vi "Logging Group Page.vi"(8 "error in (no error)":errorcluster, 11 "Node Ptr":T1 format="%.0x") -> (0 "error out":errorcluster)   [LabVIEW 2012, in "Waveform Data Logger System Explorer.lvlib"]
uses:
  Waveform Data Logger System Explorer.lvlib
  <vilib>/NI Veristand/Custom Device API/Custom Device Item Ref.ctl
  NationalInstruments.VeriStand.SystemDefinitionAPI
  NationalInstruments.VeriStand.SystemStorage
  Shared/Globals/Global GUIDs.vi
  <vilib>/NI Veristand/Custom Device Tools/Custom Device Utility Library/NI VeriStand - Search for All Items by GUID.vi
  <vilib>/NI VeriStand/Custom Device API/Custom Device API.lvlib
  <vilib>/NI VeriStand/Custom Device Tools/Custom Device Utility Library/Custom Device Utility Library.lvlib
  Shared/Waveform Data Logger Shared.lvlib
panel:
  in  "Description":string
  in  "Down Arrow":bool
  in  "Up Arrow":bool
  in  "Header 2":cluster{"Section Name":string}={"Section Name"="Waveform Log Files"}
  in  "Remove":bool
  in  "TDMS Log Files":i32(listbox)
  in  "Add File":bool
  in  "Header":cluster{"Section Name":string}={"Section Name"="Logging Group Specification"}
  in  "Name":string
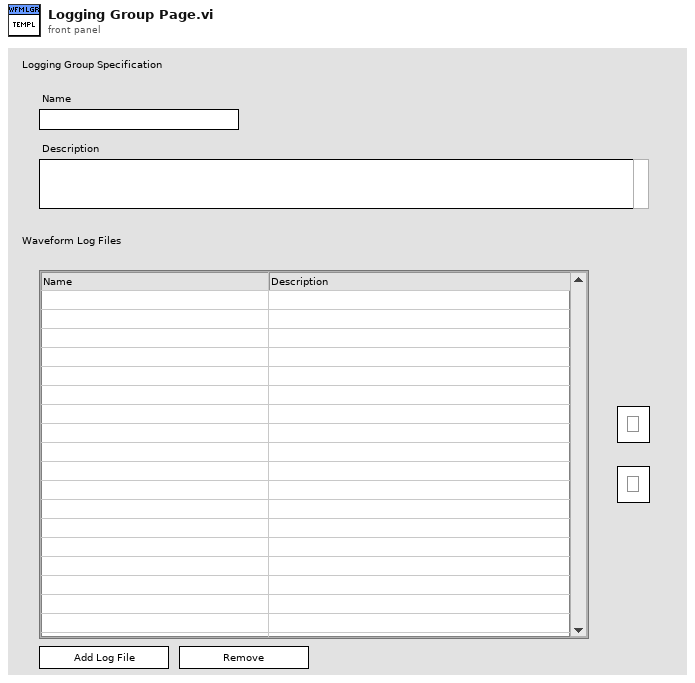
[diagram p1: front panel]
types:
  T1 = typedef "Custom Device API.lvlib/Custom Device Item Ref.ctl" = u64
  T2 = typedef "Custom Device API.lvlib/Custom Device Item Info.ctl" = cluster{"Name":string, "Is Channel":bool, "GUID":string, "Is Waveform":bool}
  T3 = typedef "Custom Device API.lvlib/Custom Device Commands.ctl" = enum16{"Default", "Item renamed", "Shutdown", "Dynamic button pressed"}
  T4 = typedef "LVRowAndColumnTypeDef.ctl" = cluster{"Row":i32, "Column":i32}
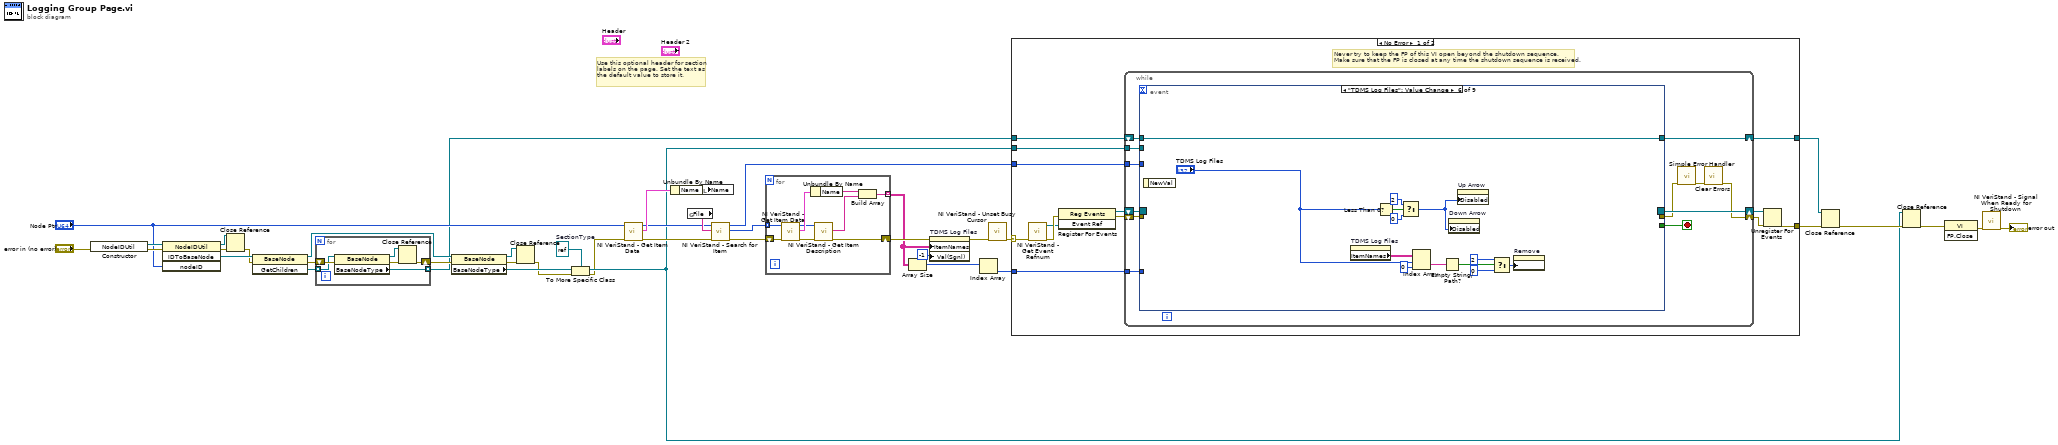
[diagram p0: block diagram]
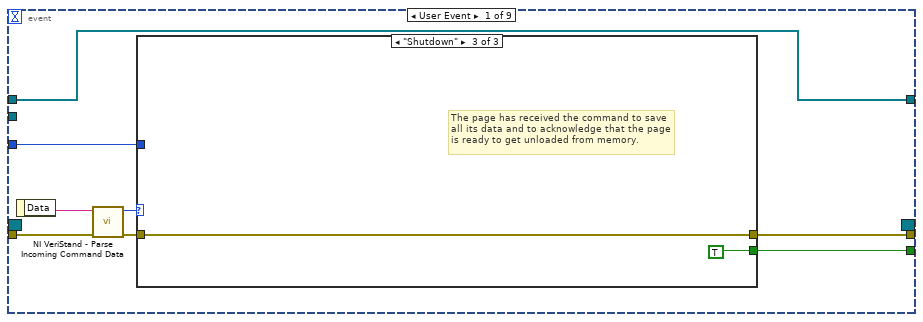
[diagram p2: hidden frame]
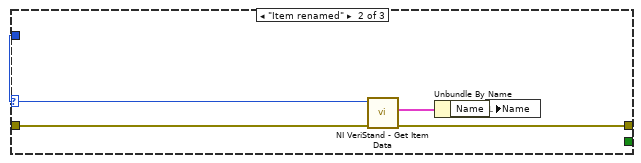
[diagram p4: hidden frame]
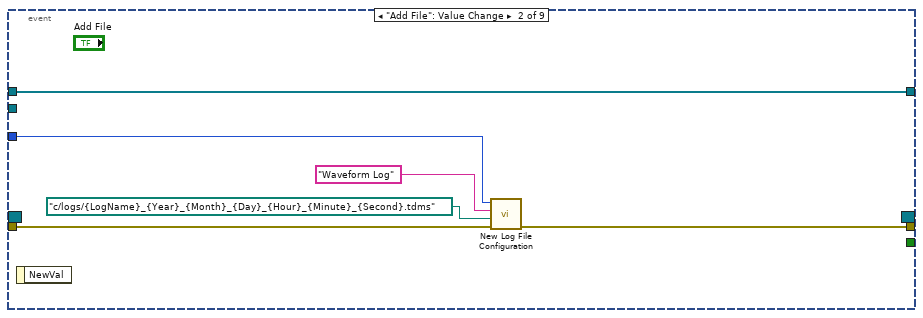
[diagram p5: hidden frame]
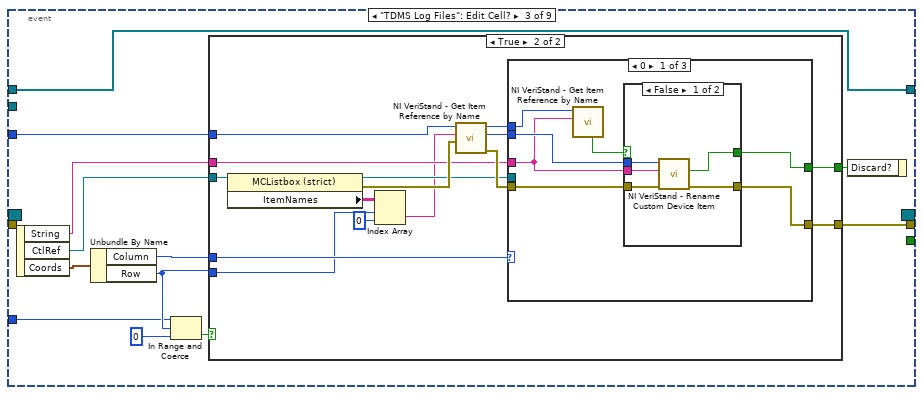
[diagram p6: hidden frame]
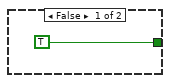
[diagram p7: hidden frame]
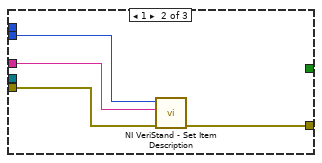
[diagram p9: hidden frame]
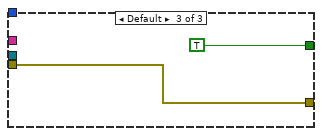
[diagram p10: hidden frame]
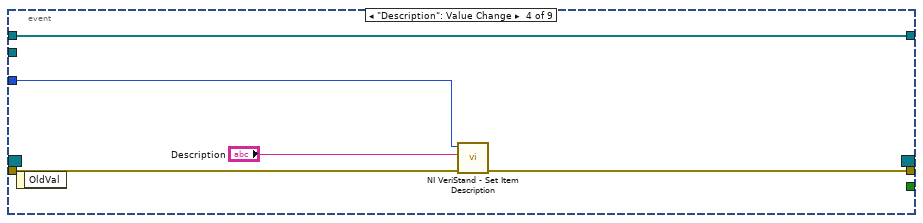
[diagram p11: hidden frame]
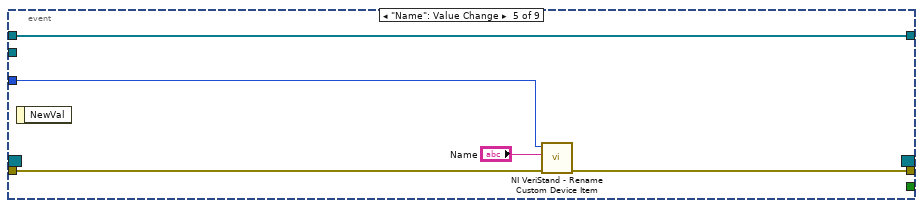
[diagram p12: hidden frame]
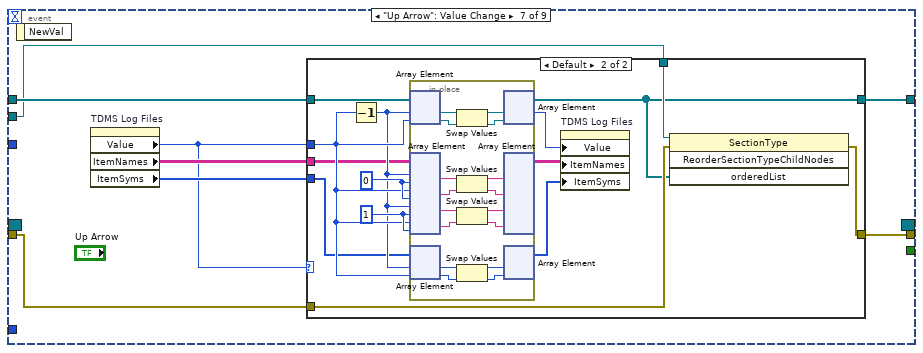
[diagram p13: hidden frame]
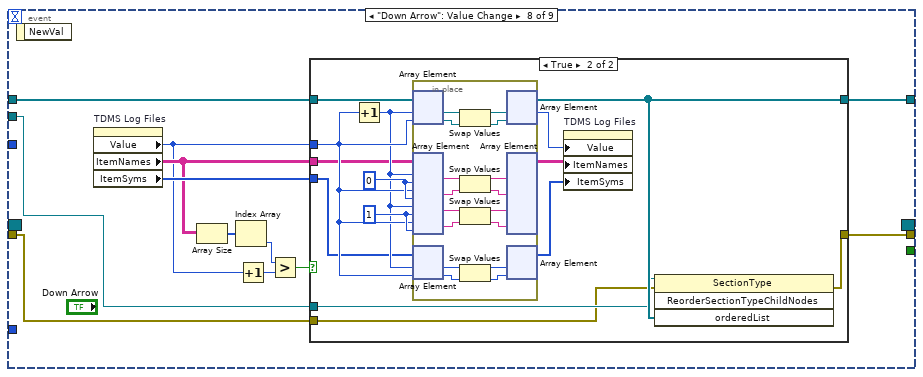
[diagram p15: hidden frame]
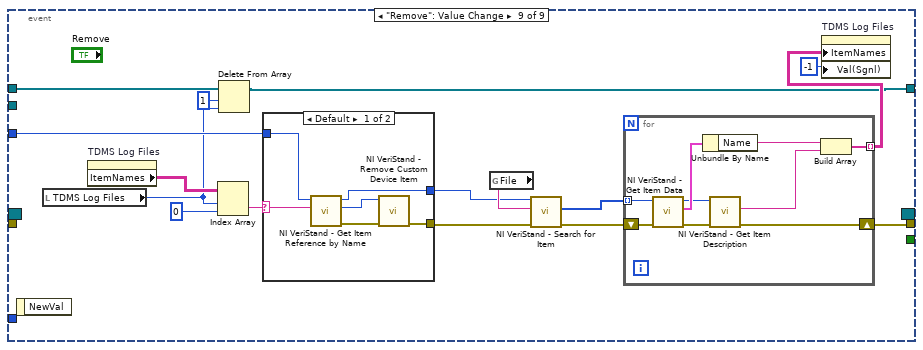
[diagram p17: hidden frame]
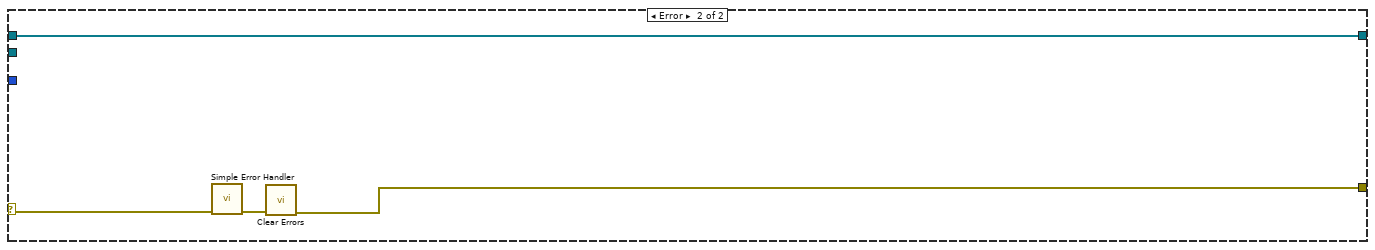
[diagram p19: hidden frame]
diagram:
  w10 = refnum<k24> refnum  # SectionType
  # "Use this optional header for section labels on the page. Set the text as the default value to store it."
  n1 = constructor class="NodeIDUtil"(error in="error in (no error)") -> (reference out=w22:refnum<k24>, error out=w23:errorcluster)  [unwired: 2 in, 1 out]
  n2 = invoke class="NodeIDUtil" method="IDToBaseNode"(reference=w22, error in=w23, "nodeID"="Node Ptr") -> (reference out=w19:refnum<k24>, error out=w24:errorcluster, "IDToBaseNode"=w18:refnum<k24>)  [unwired: 1 in, 1 out]
  n3 = Close Reference(reference=w19, error in (no error)=w24) -> (error out=w17:errorcluster)
  n4 = invoke class="BaseNode" method="GetChildren"(reference=w18, error in=w17) -> (reference out=w2:refnum<k24>, error out=w5:errorcluster, "GetChildren"=w4:refnum<k24>[])  [unwired: 1 in]
  n5 = for {
    shift-right: [w43] -> w3
    shift-left: w5 -> [w47]
    tunnel: w4 -> [w46] mode=indexing
    tunnel: [w42] -> w1 mode=indexing
    n6 = property class="BaseNode"(reference=w46, error in=w47) -> (reference out=w44:refnum<k24>, error out=w45:errorcluster, "BaseNodeType"=w42:refnum<k24>)
    n7 = Close Reference(reference=w44, error in (no error)=w45) -> (error out=w43:errorcluster)
  }
  n8 = property class="BaseNode"(reference=w2, error in=w3) -> (reference out=w15:refnum<k24>, error out=w16:errorcluster, "BaseNodeType"=w9:refnum<k24>)
  n9 = Close Reference(reference=w15, error in (no error)=w16) -> (error out=w8:errorcluster)
  n10 = To More Specific Class(target class=w10, reference=w9, error in=w8) -> (specific class reference=w7:refnum<k24>, error out=w6:errorcluster)
  n11 = call <vilib>:"NI VeriStand - Get Item Data.vi"("error in (no error)"=w6, "Item Ref in"="Node Ptr") -> ("error out"=w25:errorcluster, "Item Info"=w38:T2, "Item Ref out"=w26:T1)  [unwired: 7 out]
  n12 = Unbundle By Name(w38) -> ("Name"=w37:string)
  n13 = global read "Global GUIDs.vi" "File"() -> (w27:string)
  n14 = local write "Name"(w37) -> ()
  n15 = call-poly <vilib>:"NI VeriStand - Search for Item.vi"("error in"=w25, "Item GUID"=w27, "Section Ref in"=w26) -> ("error out"=w30:errorcluster, "Item Refs"=w29:T1[], "Section Ref out"=w28:T1)  [unwired: 5 in, 1 out]
  n16 = for {
    tunnel: w29 -> [w55] mode=indexing
    tunnel: [w51] -> w33 mode=indexing
    shift-right: [w50] -> w36
    shift-left: w30 -> [w56]
    n17 = call <vilib>:"NI VeriStand - Get Item Data.vi"("error in (no error)"=w56, "Item Ref in"=w55) -> ("error out"=w48:errorcluster, "Item Info"=w54:T2, "Item Ref out"=w49:T1)  [unwired: 6 in, 1 out]
    n18 = Unbundle By Name(w54) -> ("Name"=w53:string)
    n19 = call <vilib>:"NI VeriStand - Get Item Description.vi"("error in (no error)"=w48, "Item Ref in"=w49) -> ("error out"=w50:errorcluster, "Description"=w52:string)  [unwired: 6 in, 2 out]
    n20 = Build Array(w53, w52) -> (w51:string[])
  }
  n21 = Array Size(array=w33) -> (size(s)=w32:i32[])
  n22 = property on="TDMS Log Files" class="MCListbox (strict)"(error in=w36, "ItemNames"=w33, "Val(Sgnl)"=-1 ("Value (Signaling)")) -> (error out=w34:errorcluster)  [unwired: 1 in, 1 out]
  n23 = Index Array(array=w32) -> (element=w31:i32)  [unwired: 1 in]
  n24 = call <vilib>:"NI VeriStand - Unset Busy Cursor.vi"("error in (no error)"=w34) -> ("error out"=w39:errorcluster)  [unwired: 10 out]
  n25 = case shown="No Error" w39 {
    selector: w39 -> [w62 w294]
    tunnel: [w57 w292] -> w13
    tunnel: w28 -> [w63 _]
    tunnel: w31 -> [w61 _]
    tunnel: w1 -> [w60 w291]
    tunnel: w7 -> [w59 _]
    tunnel: [w58 w291] -> w12
    frame No Error {
      # "Never try to keep the FP of this VI open beyond the shutdown sequence.\nMake sure that the FP is closed at any time the shutdown sequence is received."
      n26 = call <vilib>:"NI VeriStand - Get Event Refnum.vi"("error in (no error)"=w62) -> ("error out"=w69:errorcluster, "Event Ref"=w66:refnum<user-event>)  [unwired: 9 out]
      n27 = register-events(error in=w69, w66) -> (reference out=w64:refnum<event-registration>, error out=w65:errorcluster)  [unwired: 1 in]
      n28 = while {
        tunnel: w63 -> [w78]
        shift-right: [w75] -> w67
        shift-left: w65 -> [w80]
        shift-right: [w81] -> w68
        shift-left: w64 -> [w73]
        tunnel: w61 -> [w74]
        shift-right: [w71] -> w58
        shift-left: w60 -> [w72]
        tunnel: w59 -> [w70]
        stop <- w79 stop-if-true
        n29 = event shown="[5] \"TDMS Log Files\": Value Change" {
          selector: w73 -> [_ _ _ _ _ _ _ _ _]
          dyn-events: [_ _ _ _ _ _ _ _ _] -> w81
          timeout: _ -> [_ _ _ _ _ _ _ _ _]
          tunnel: w80 -> [w89 w102 _ w156 w161 _ w176 w217 _]
          tunnel: [w85 _ _ _ _ _ _ _ _] -> w79
          tunnel: [w84 w101 w111 w153 w160 _ w175 w216 w265] -> w77
          tunnel: w78 -> [w83 w103 w106 w154 w159 _ _ _ w272]
          tunnel: w74 -> [_ _ w105 _ _ _ _ _ _]
          tunnel: w72 -> [w82 w98 w104 w152 w157 w170 w179 w219 w262]
          tunnel: [w82 w98 w104 w152 w157 w170 w178 w215 w259] -> w71
          tunnel: w70 -> [_ _ _ _ _ _ w177 w218 _]
          event User Event {
            n30 = event-data() -> ("Data"=w88:string)  [unwired: 1 out]
            n31 = call <vilib>:"NI VeriStand - Parse Incoming Command Data.vi"("error in (no error)"=w89, "Incoming data"=w88) -> ("error out"=w87:errorcluster, "Action"=w86:T3)  [unwired: 8 out]
            n32 = case shown="\"Shutdown\"" w86 {
              tunnel: w87 -> [w90 w95 w96]
              tunnel: [_ _ TRUE] -> w85
              tunnel: [w90 w92 w96] -> w84
              tunnel: w83 -> [_ w94 _]
              frame "Default", Default {
              }
              frame "Item renamed" {
                n33 = call <vilib>:"NI VeriStand - Get Item Data.vi"("error in (no error)"=w95, "Item Ref in"=w94) -> ("error out"=w92:errorcluster, "Item Info"=w93:T2)  [unwired: 8 out]
                n34 = Unbundle By Name(w93) -> ("Name"=w91:string)
                n35 = local write "Name"(w91) -> ()
              }
              frame "Shutdown" {
                # "The page has received the command to save all its data and to acknowledge that the page is ready to get unloaded from memory."
              }
            }
          }
          event "Add File": Value Change {
            n36 = event-data() -> ()  [unwired: 2 out]
            n37 = call "New Log File Configuration.vi"("error in (no error)"=w102, "Default Path"=path "c:/logs/{LogName}_{Year}_{Month}_{Day}_{Hour}_{Minute}_{Second}.tdms" ("Default Log Directory"), "Default Name"="Waveform Log", "Device Ref in"=w103) -> ("error out"=w101:errorcluster)  [unwired: 7 out]
          }
          event "TDMS Log Files": Edit Cell? {
            n38 = event-data() -> ("String"=w108:string, "CtlRef"=w107:refnum<vi>, "Coords"=w109:T4)  [unwired: 1 out]
            n39 = Unbundle By Name(w109) -> ("Column"=w115:i32, "Row"=w113:i32)
            n40 = In Range and Coerce(upper limit=w105, x=w113, lower limit=0) -> (In Range?=w112:bool)  [unwired: 1 out]
            n41 = case shown="True" w112 {
              tunnel: w107 -> [_ w129]
              tunnel: [TRUE w126] -> w110
              tunnel: w108 -> [_ w124]
              tunnel: w106 -> [_ w122]
              tunnel: w113 -> [_ w121]
              tunnel: w115 -> [_ w127]
              tunnel: [_ w123] -> w111
              frame False {
              }
              frame True {
                n42 = property class="MCListbox (strict)"(reference=w129) -> (reference out=w125:refnum<vi>, error out=w131:errorcluster, "ItemNames"=w128:string[][])  [unwired: 1 in]
                n43 = Index Array(array=w128, index (row)=w121, index (col)=0 ("disabled index (col)")) -> (element=w119:string)
                n44 = call <vilib>:"NI VeriStand - Get Item Reference by Name.vi"("error in (no error)"=w131, "Item Name"=w119, "Parent Ref in"=w122) -> ("error out"=w130:errorcluster, "Item Ref"=w118:T1, "Parent Ref out"=w117:T1)  [unwired: 5 in, 1 out]
                n45 = case shown="0" w127 {
                  tunnel: [w132 _ TRUE] -> w126
                  tunnel: w118 -> [w137 w148 _]
                  tunnel: w130 -> [w138 w146 w150]
                  tunnel: w125 -> [_ _ _]
                  tunnel: w124 -> [w134 w147 _]
                  tunnel: [w136 w149 w150] -> w123
                  tunnel: w117 -> [w135 _ _]
                  frame 0 {
                    n46 = call <vilib>:"NI VeriStand - Get Item Reference by Name.vi"("Item Name"=w134, "Parent Ref in"=w135) -> ("Found"=w133:bool)  [unwired: 6 in, 3 out]
                    n47 = case shown="False" w133 {
                      selector: w133 -> [_ w144]
                      tunnel: w138 -> [w143 w145]
                      tunnel: w137 -> [w142 _]
                      tunnel: [w141 w145] -> w136
                      tunnel: w134 -> [w140 _]
                      tunnel: [w139 w144] -> w132
                      frame False {
                        n48 = call <vilib>:"NI VeriStand - Rename Custom Device Item.vi"("error in (no error)"=w143, "New Name"=w140, "Item Ref in"=w142) -> ("error out"=w141:errorcluster, "Request invalid?"=w139:bool)  [unwired: 6 in, 1 out]
                      }
                      frame True {
                        # "Ignore. File\nby that name\nalready exists."
                      }
                    }
                  }
                  frame 1 {
                    n49 = call <vilib>:"NI VeriStand - Set Item Description.vi"("error in (no error)"=w146, "Description"=w147, "Item Ref in"=w148) -> ("error out"=w149:errorcluster)  [unwired: 6 in, 2 out]
                  }
                  frame Default {
                  }
                }
              }
            }
            n50 = event-data("Discard?"=w110) -> ()  [unwired: 1 in, 1 out]
          }
          event "Description": Value Change {
            n51 = event-data() -> ()  [unwired: 2 out]
            n52 = call <vilib>:"NI VeriStand - Set Item Description.vi"("error in (no error)"=w156, "Description"="Description", "Item Ref in"=w154) -> ("error out"=w153:errorcluster)  [unwired: 8 out]
          }
          event "Name": Value Change {
            n53 = event-data() -> ()  [unwired: 2 out]
            n54 = call <vilib>:"NI VeriStand - Rename Custom Device Item.vi"("error in (no error)"=w161, "New Name"="Name", "Item Ref in"=w159) -> ("error out"=w160:errorcluster)  [unwired: 1 in, 7 out]
          }
          event "TDMS Log Files": Value Change {
            n55 = event-data() -> ()  [unwired: 2 out]
            n56 = property on="TDMS Log Files" class="MCListbox (strict)"() -> ("ItemNames"=w163:string[][])  [unwired: 2 in, 2 out]
            n57 = Less Than 0?(x="TDMS Log Files") -> (x < 0?=w171:bool)
            n58 = Select(t=u8 2 ("Disabled"), s=w171, f=u8 0 ("Disabled")) -> (s? t:f=w174:u8)
            n59 = Index Array(array=w163, index (row)="TDMS Log Files", index (col)=0 ("disabled index (col)")) -> (element=w166:string)
            n60 = Empty String/Path?(string/path=w166) -> (empty?=w165:bool)
            n61 = property on="Down Arrow" class="Bool"("Disabled"=w174) -> ()  [unwired: 2 in, 2 out]
            n62 = property on="Up Arrow" class="Bool"("Disabled"=w174) -> ()  [unwired: 2 in, 2 out]
            n63 = Select(t=u8 2, s=w165, f=u8 0) -> (s? t:f=w167:u8)
            n64 = property on="Remove" class="Bool"("DisabledEnum"=w167) -> ()  [unwired: 2 in, 2 out]
          }
          event "Up Arrow": Value Change {
            n65 = event-data() -> ()  [unwired: 2 out]
            n66 = property on="TDMS Log Files" class="MCListbox (strict)"() -> ("Value"=w180:i32, "ItemNames"=w181:string[][], "ItemSyms"=w182:i32[])  [unwired: 2 in, 2 out]
            n67 = case shown="Default" w180 {
              tunnel: w179 -> [w184 w198]
              tunnel: [w184 w185] -> w178
              tunnel: w180 -> [_ w193]
              tunnel: w181 -> [_ w190]
              tunnel: w182 -> [_ w189]
              tunnel: w177 -> [_ w188]
              tunnel: w176 -> [w183 w187]
              tunnel: [w183 w186] -> w175
              frame 0 {
              }
              frame Default {
                w195 = 1
                w196 = 0
                n68 = Decrement(x=w193) -> (x-1=w192:i32)
                n69 = in-place {
                  n70 = in-place-array #1(w198, w192, w193) -> (w214:refnum<k24>, w213:refnum<k24>)
                  n71 = in-place-array #2(w190, w192, w196, w193, w196, w192, w195, w193, w195) -> (w210:string, w209:string, w206:string, w205:string)
                  n72 = in-place-array #3(w189, w192, w193) -> (w202:i32, w201:i32)
                  n73 = Swap Values(12:w214, 14:w213) -> (1:w212:refnum<k24>, 3:w211:refnum<k24>)  [unwired: 1 out]
                  n74 = Swap Values(12:w210, 14:w209) -> (1:w208:string, 3:w207:string)  [unwired: 1 out]
                  n75 = Swap Values(12:w206, 14:w205) -> (1:w204:string, 3:w203:string)  [unwired: 1 out]
                  n76 = Swap Values(12:w202, 14:w201) -> (1:w200:i32, 3:w199:i32)  [unwired: 1 out]
                  n77 = in-place-array #1(w212, w211) -> (w185:refnum<k24>[], w194:i32)  [unwired: 1 out]
                  n78 = in-place-array #2(w208, w207, w204, w203) -> (w197:string[][])  [unwired: 8 out]
                  n79 = in-place-array #3(w200, w199) -> (w191:i32[])  [unwired: 2 out]
                }
                n80 = property on="TDMS Log Files" class="MCListbox (strict)"("Value"=w194, "ItemNames"=w197, "ItemSyms"=w191) -> ()  [unwired: 2 in, 2 out]
                n81 = invoke class="SectionType" method="ReorderSectionTypeChildNodes"(reference=w188, error in=w187, "orderedList"=w185) -> (error out=w186:errorcluster)  [unwired: 1 in, 3 out]
              }
            }
          }
          event "Down Arrow": Value Change {
            n82 = event-data() -> ()  [unwired: 2 out]
            n83 = property on="TDMS Log Files" class="MCListbox (strict)"() -> ("Value"=w220:i32, "ItemNames"=w225:string[][], "ItemSyms"=w226:i32[])  [unwired: 2 in, 2 out]
            n84 = Array Size(array=w225) -> (size(s)=w222:i32[])
            n85 = Index Array(array=w222) -> (element=w223:i32)  [unwired: 1 in]
            n86 = Increment(x=w220) -> (x+1=w221:i32)
            n87 = Greater?(x=w223, y=w221) -> (0:w224:bool)
            n88 = case shown="True" w224 {
              tunnel: w219 -> [w228 w242]
              tunnel: [w228 w232] -> w215
              tunnel: w220 -> [_ w237]
              tunnel: w225 -> [_ w234]
              tunnel: w226 -> [_ w233]
              tunnel: w218 -> [_ w231]
              tunnel: w217 -> [w227 w230]
              tunnel: [w227 w229] -> w216
              frame False {
              }
              frame True {
                w239 = 1
                w240 = 0
                n89 = Increment(x=w237) -> (x+1=w236:i32)
                n90 = in-place {
                  n91 = in-place-array #4(w242, w236, w237) -> (w258:refnum<k24>, w257:refnum<k24>)
                  n92 = in-place-array #5(w234, w236, w240, w237, w240, w236, w239, w237, w239) -> (w254:string, w253:string, w250:string, w249:string)
                  n93 = in-place-array #6(w233, w236, w237) -> (w246:i32, w245:i32)
                  n94 = Swap Values(12:w258, 14:w257) -> (1:w256:refnum<k24>, 3:w255:refnum<k24>)  [unwired: 1 out]
                  n95 = Swap Values(12:w254, 14:w253) -> (1:w252:string, 3:w251:string)  [unwired: 1 out]
                  n96 = Swap Values(12:w250, 14:w249) -> (1:w248:string, 3:w247:string)  [unwired: 1 out]
                  n97 = Swap Values(12:w246, 14:w245) -> (1:w244:i32, 3:w243:i32)  [unwired: 1 out]
                  n98 = in-place-array #4(w256, w255) -> (w232:refnum<k24>[], w238:i32)  [unwired: 1 out]
                  n99 = in-place-array #5(w252, w251, w248, w247) -> (w241:string[][])  [unwired: 8 out]
                  n100 = in-place-array #6(w244, w243) -> (w235:i32[])  [unwired: 2 out]
                }
                n101 = property on="TDMS Log Files" class="MCListbox (strict)"("Value"=w238, "ItemNames"=w241, "ItemSyms"=w235) -> ()  [unwired: 2 in, 2 out]
                n102 = invoke class="SectionType" method="ReorderSectionTypeChildNodes"(reference=w231, error in=w230, "orderedList"=w232) -> (error out=w229:errorcluster)  [unwired: 1 in, 3 out]
              }
            }
          }
          event "Remove": Value Change {
            n103 = event-data() -> ()  [unwired: 2 out]
            n104 = local read "TDMS Log Files"() -> (w261:i32)
            n105 = property on="TDMS Log Files" class="MCListbox (strict)"() -> ("ItemNames"=w271:string[][])  [unwired: 2 in, 2 out]
            n106 = Index Array(array=w271, index (row)=w261, index (col)=0 ("disabled index (col)")) -> (element=w274:string)
            n107 = Delete From Array(array=w262, length=1, index=w261) -> (array with subset deleted=w259:refnum<k24>[])  [unwired: 1 out]
            n108 = case shown="Default" w274 {
              selector: w274 -> [w286 _]
              tunnel: w272 -> [w287 w290]
              tunnel: [w289 _] -> w264
              tunnel: [w284 w290] -> w263
              frame Default {
                n109 = call <vilib>:"NI VeriStand - Get Item Reference by Name.vi"("Item Name"=w286, "Parent Ref in"=w287) -> ("error out"=w288:errorcluster, "Item Ref"=w285:T1, "Parent Ref out"=w284:T1)  [unwired: 6 in, 1 out]
                n110 = call <vilib>:"NI VeriStand - Remove Custom Device Item.vi"("error in (no error)"=w288, "Item Ref in"=w285) -> ("error out"=w289:errorcluster)  [unwired: 8 in, 1 out]
              }
              frame "" {
              }
            }
            n111 = global read "Global GUIDs.vi" "File"() -> (w268:string)
            n112 = call-poly <vilib>:"NI VeriStand - Search for Item.vi"("error in"=w264, "Item GUID"=w268, "Section Ref in"=w263) -> ("error out"=w270:errorcluster, "Item Refs"=w269:T1[])  [unwired: 5 in, 2 out]
            n113 = for {
              tunnel: w269 -> [w282] mode=indexing
              tunnel: [w278] -> w266 mode=indexing
              shift-right: [w277] -> w265
              shift-left: w270 -> [w283]
              n114 = call <vilib>:"NI VeriStand - Get Item Data.vi"("error in (no error)"=w283, "Item Ref in"=w282) -> ("error out"=w275:errorcluster, "Item Info"=w281:T2, "Item Ref out"=w276:T1)  [unwired: 6 in, 1 out]
              n115 = Unbundle By Name(w281) -> ("Name"=w280:string)
              n116 = call <vilib>:"NI VeriStand - Get Item Description.vi"("error in (no error)"=w275, "Item Ref in"=w276) -> ("error out"=w277:errorcluster, "Description"=w279:string)  [unwired: 6 in, 2 out]
              n117 = Build Array(w280, w279) -> (w278:string[])
            }
            n118 = property on="TDMS Log Files" class="MCListbox (strict)"("ItemNames"=w266, "Val(Sgnl)"=-1 ("Value (Signaling)")) -> ()  [unwired: 2 in, 2 out]
          }
        }
        n119 = call <vilib>:"Simple Error Handler.vi"("error in (no error)"=w77) -> ("error out"=w76:errorcluster)  [unwired: 1 in, 7 out]
        n120 = call <vilib>:"Clear Errors.vi"("error in (no error)"=w76) -> ("error out"=w75:errorcluster)  [unwired: 6 out]
      }
      n121 = Unregister For Events(event registration refnum=w68, error in=w67) -> (error out=w57:errorcluster)
    }
    frame Error {
      n122 = call <vilib>:"Simple Error Handler.vi"("error in (no error)"=w294) -> ("error out"=w293:errorcluster)  [unwired: 1 in, 7 out]
      n123 = call <vilib>:"Clear Errors.vi"("error in (no error)"=w293) -> ("error out"=w292:errorcluster)  [unwired: 6 out]
    }
  }
  n124 = Close Reference(reference=w12, error in (no error)=w13) -> (error out=w11:errorcluster)
  n125 = Close Reference(reference=w7, error in (no error)=w11) -> (error out=w14:errorcluster)
  n126 = invoke class="VI" method="FP.Close"(error in=w14) -> (error out=w41:errorcluster)  [unwired: 2 in, 2 out]
  n127 = call <vilib>:"NI VeriStand - Signal When Ready for Shutdown.vi"("error in (no error)"=w41) -> ("error out"=→"error out":errorcluster)  [unwired: 10 out]
